vi "Get_X_constraints.vi"(8 "error in (no error)":errorcluster, 11 "FAMM in":refnum<class "FAMM.lvclass">) -> (0 "error out":errorcluster, 2 "X-constraints":T1, 3 "FAMM out":refnum<class "FAMM.lvclass">)   [LabVIEW 2020, in "Sgraph_lib_V1.lvlib" / "FAMM.lvclass"]
doc: "Get X-constraints"
uses:
  FAMM.lvclass
  controls/FAMM_reply_X-axis-constraints.ctl
  FAMM.lvclass/FAMM.ctl
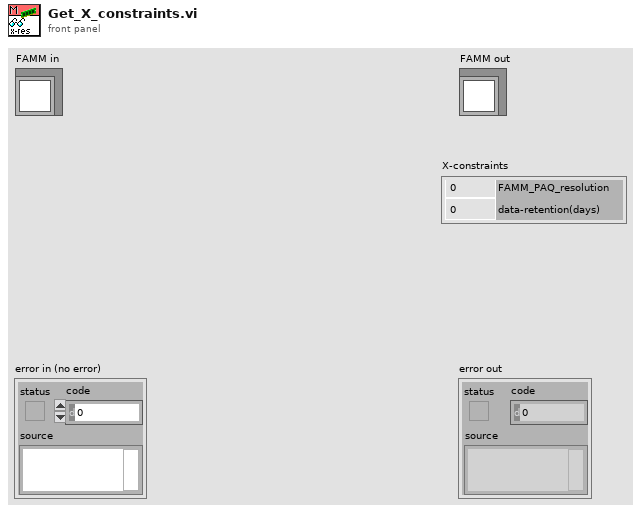
[diagram p1: front panel]
types:
  T1 = cluster{"FAMM_PAQ_resolution":dbl, "data-retention(days)":dbl}
  T2 = typedef "Sgraph_lib_V1.lvlib/FAMM.lvclass/FAMM_reply_X-axis-constraints.ctl" = cluster{"FAMM_PAQ_resolution":dbl, "data-retention(days)":dbl}
  T3 = typedef "Sgraph_lib_V1.lvlib/FAMM.lvclass/FAMM-attributes.ctl" = cluster{"FAMM_PAQ_Layers":i32, "FAMM_PAQ_resolution":dbl, "PAQ_TAGs":string[], "WAQ_TAGs":string[], "EAQ_TAGs":string[], "All_TAGs":string[], "PAQtagProps":T4[], "WAQtagProps":T4[], "EAQtagProps":T4[], "DBAL_class":refnum<data-value>, "PAQ_memory":refnum<data-value>[], "PAQupdates":timestamp[], "FAMM_Size":cluster{"other":i32, "1day":i32, "1week":i32}, "DatabaseFileExtention":string, "DatabaseSaveRate":dbl, "Database_path":path, "DBAL-Queue":refnum<queue>, "OS_name":string, "ini-file":string, "data-retention(days)":dbl}
  T4 = typedef "Sgraph_lib_V1.lvlib/typedef_com_TagProp.ctl" = cluster{"Description":string, "EngUnits":string, "RangeH":dbl, "RangeL":dbl, "Resolution":i32, "Obsolete":bool, "ChangeDate":timestamp, "ChangeSource":string, "ChangeReason":string, "TagFunc":u32}
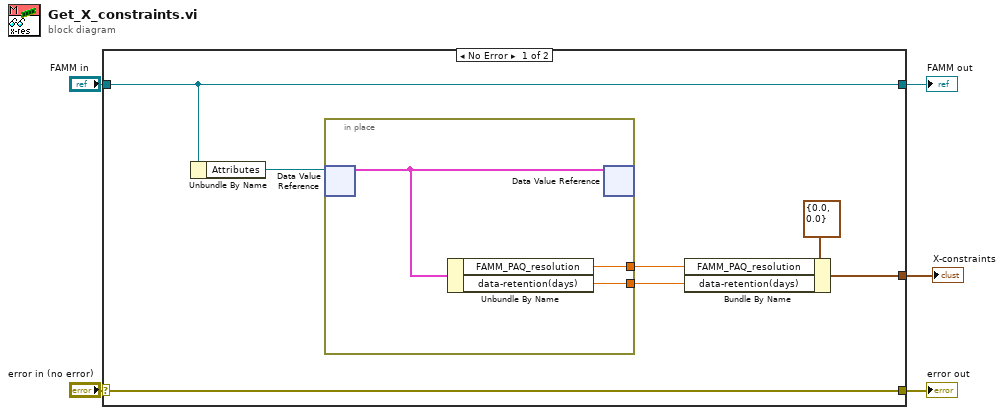
[diagram p0: block diagram]
diagram:
  n1 = case shown="No Error" "error in (no error)" {
    selector: "error in (no error)" -> [w12 w16]
    tunnel: [w12 w16] -> w4
    tunnel: [w11 w17] -> w2
    tunnel: "FAMM in" -> [w11 w17]
    tunnel: [w6 _] -> w1
    frame No Error {
      n2 = Unbundle By Name(w11) -> ("Attributes"=w10:refnum<data-value>)
      n3 = in-place {
        in-place-border: [w14] -> w8
        in-place-border: [w13] -> w7
        n4 = in-place-dvr #1(w10) -> (w15:T3)  [unwired: 1 out]
        n5 = Unbundle By Name(w15) -> ("FAMM_PAQ_resolution"=w14:dbl, "data-retention(days)"=w13:dbl)
        n6 = in-place-dvr #1(w15) -> ()  [unwired: 2 out]
      }
      n7 = Bundle By Name(cluster=T2 {"FAMM_PAQ_resolution"=0.0, "data-retention(days)"=0.0} ("X-constraints"), "FAMM_PAQ_resolution"=w8, "data-retention(days)"=w7) -> (w6:T2)
    }
    frame Error {
    }
  }
  "error out" <- w4
  "FAMM out" <- w2
  "X-constraints" <- w1
